vi "Replace Array Subset.vi"() -> ()   [LabVIEW 2017]
panel:
  out "Output Array":string[](array[string])
  in  "Index":i32=2
  in  "New Element":string
  in  "Array":string[](array[string])
  # "Replace Array Subset Example"
  # "Takes New Element and replaces\nan element in the array based\non the input Index"
  # "Note that if Index\nis greater or less than\nthe number of Elements,\nnothing will happen."
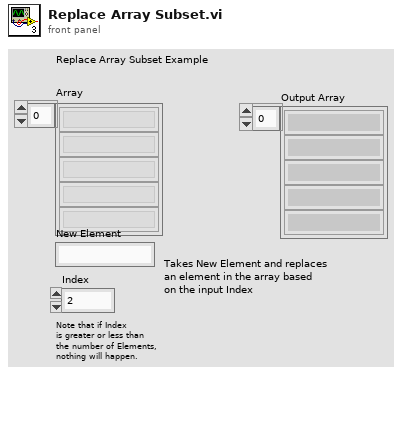
[diagram p1: front panel]
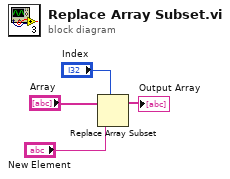
[diagram p0: block diagram]
diagram:
  n1 = Replace Array Subset(array="Array", new element="New Element", index="Index") -> (→"Output Array":string[])
